vi "TTA_MATLAB_TxACPRTest.vi"(0 "Sub-Function Name":string, 1 "Instrument Cluster In":T3, 5 "Test Group":string, 11 "error in":errorcluster) -> (4 "SubTestSuccess":dbl[](array[numeric]), 12 "Instrument Cluster Out":T3, 15 "error out":errorcluster)   [LabVIEW 2016]
uses:
  TTA_Controls/TTA_Control_Complete_Settings_Cluster.ctl
  TTA_Controls/TTA_Control_Instrument_Cluster.ctl
  TTA_Globals/TTA_Global_Complete_Settings.vi
panel:
  out "Active ACPR Cluster":T1
  out "Channel":string
  out "Tx":string
  out "ACPR Results":T2(array[cluster])
  out "Test Status":string
  in  "Complete Settings Cluster":T4
  out "RFICs":i32[](array[numeric])
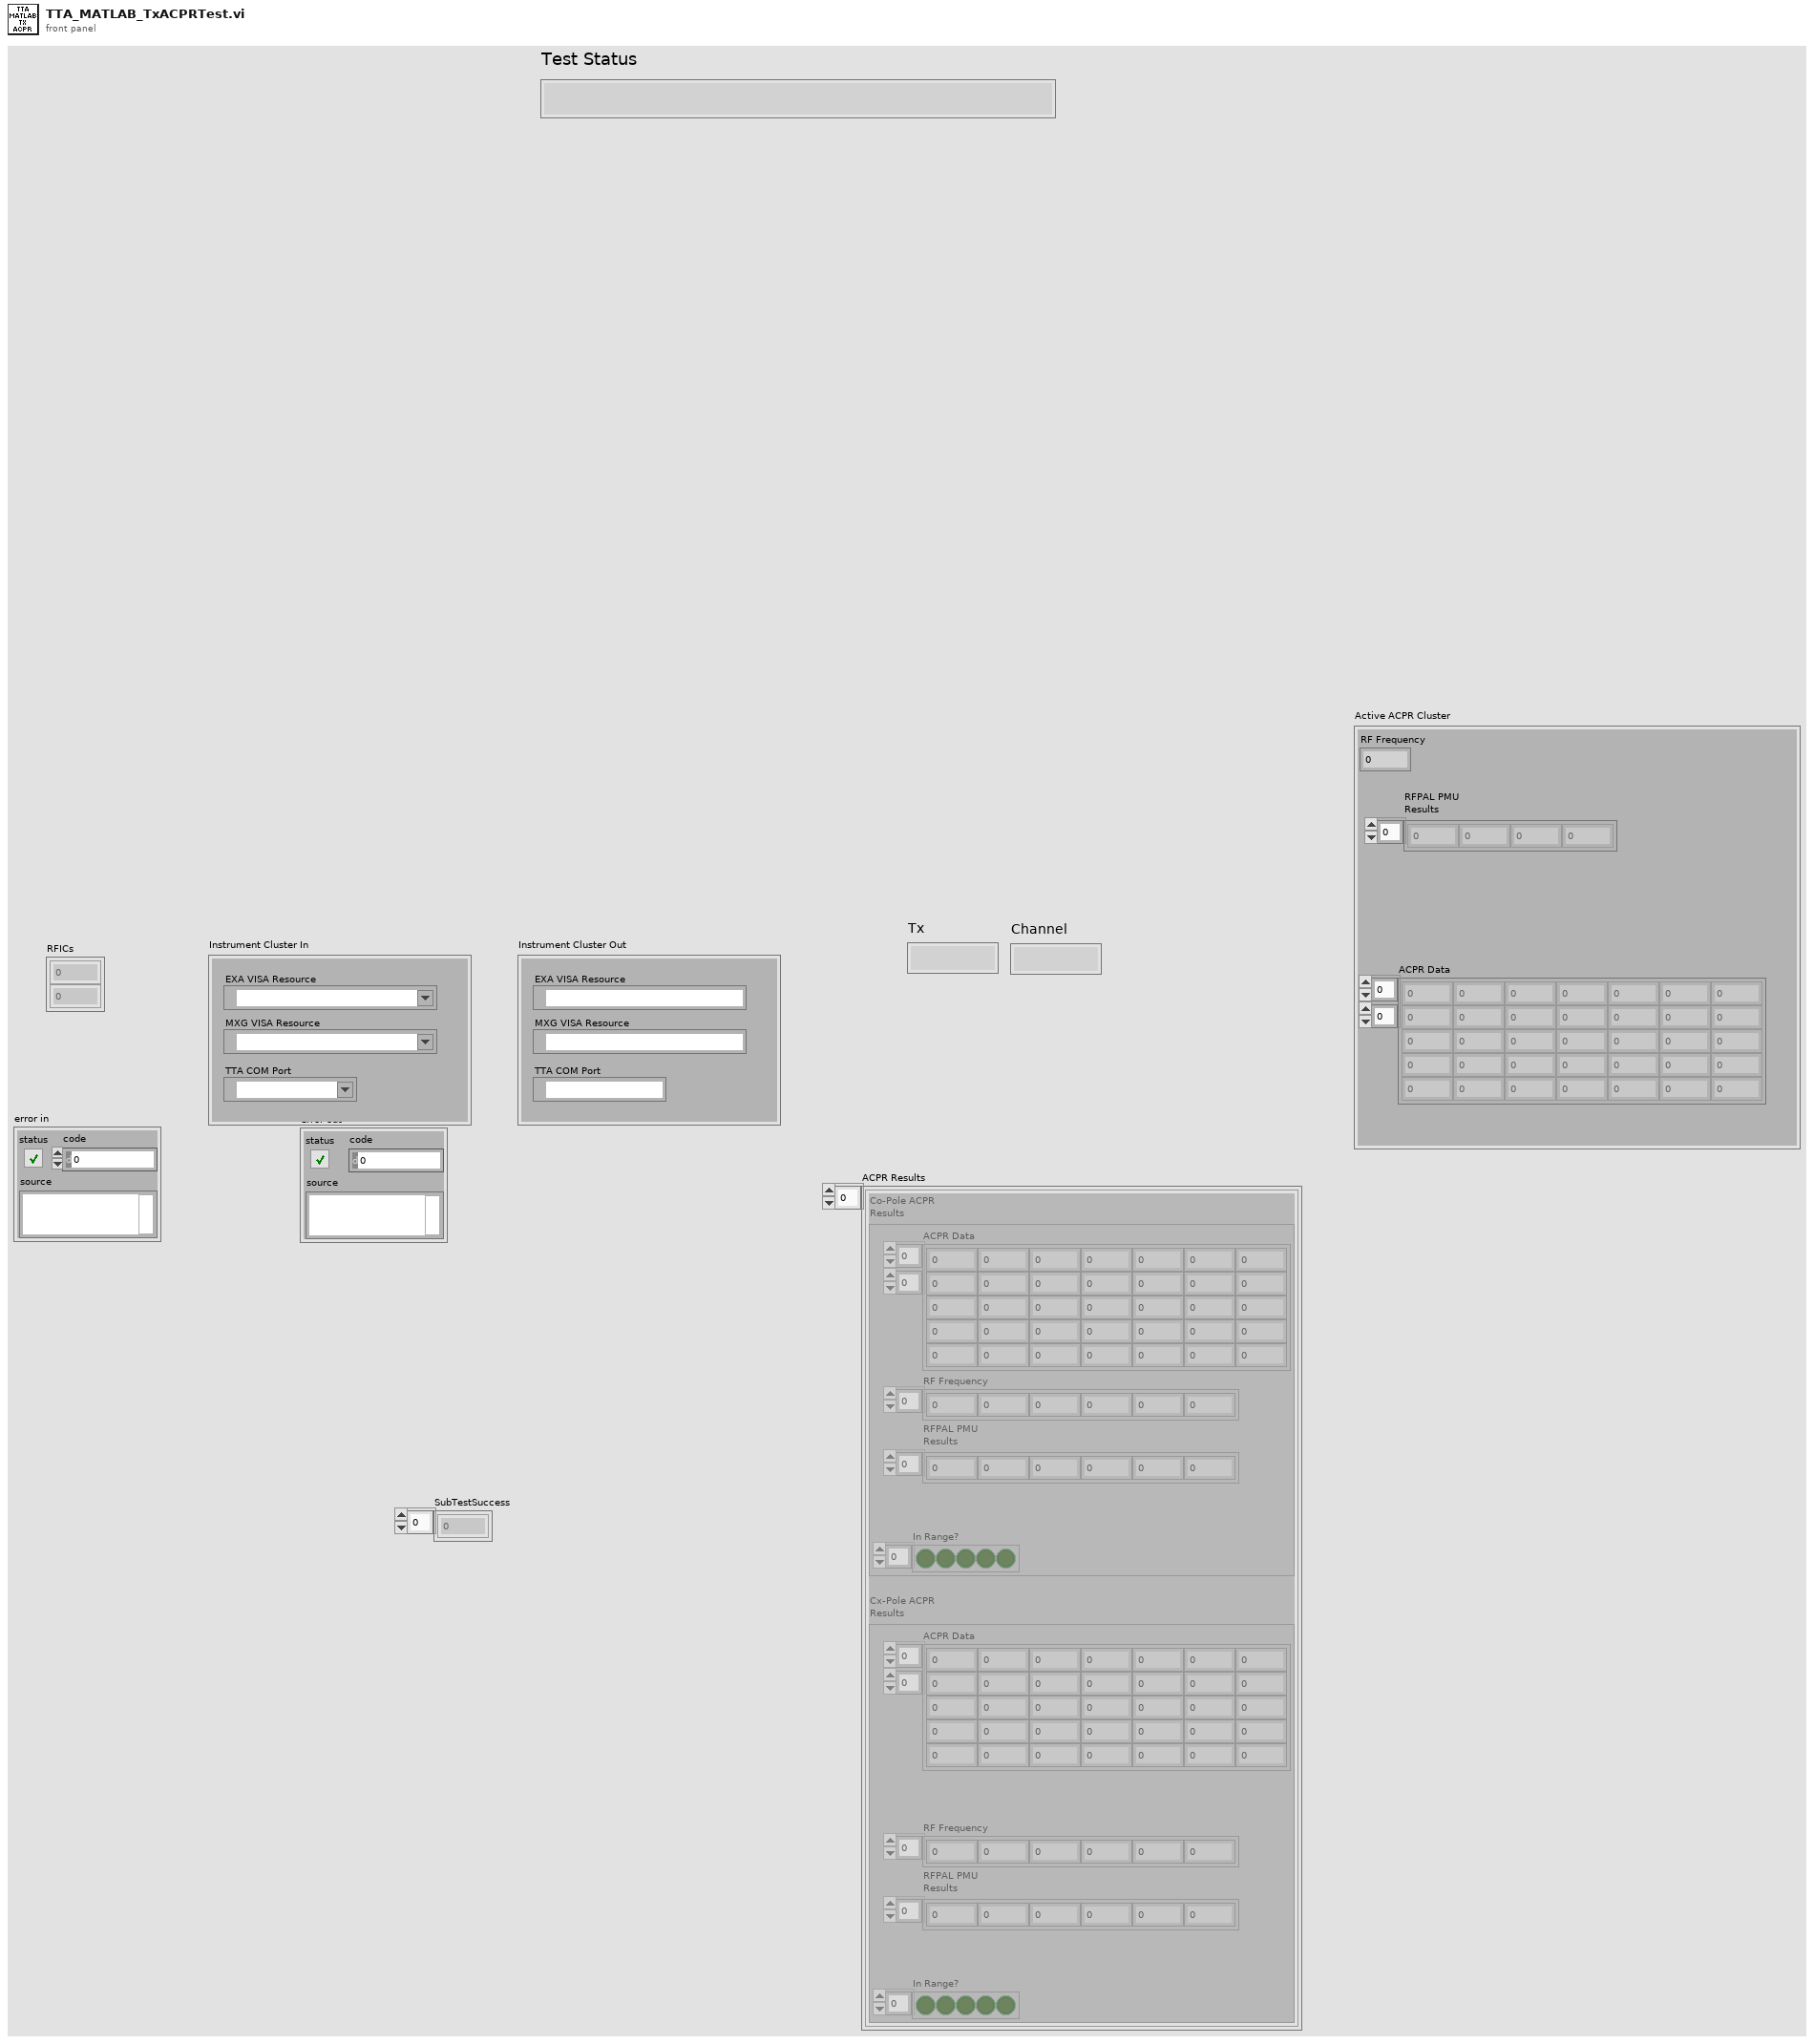
[diagram p1: front panel]
types:
  T1 = cluster{"RF Frequency":dbl, "RFPAL PMU\nResults":dbl[], "ACPR Data ":dbl[][]}
  T2 = cluster{"Co-Pole ACPR\nResults":cluster{"ACPR Data":dbl[][], "RF Frequency":dbl[], "RFPAL PMU\nResults":dbl[], "In Range?":bool[]}, "Cx-Pole ACPR\nResults":cluster{"ACPR Data":dbl[][], "RF Frequency":dbl[], "RFPAL PMU\nResults":dbl[], "In Range?":bool[]}}[]
  T3 = typedef "TTA_Control_Instrument_Cluster.ctl" = cluster{"EXA VISA Resource":refnum<visa-resource-name>, "MXG VISA Resource":refnum<visa-resource-name>, "TTA COM Port":refnum<visa-resource-name>}
  T4 = typedef "TTA_Control_Complete_Settings_Cluster.ctl" = cluster{"Brief Cluster":cluster{"STM Firmware File":string, "STM Firmware Address":string, "Required SW Version":string, "Template Used":string}, "Instrument Setting Cluster":cluster{"BDSFreq":dbl, "BDS Amp":dbl, "TxRFCal_Freq":dbl, "TxRFCal_Amp":dbl, "RxRFCal_Freq":dbl, "RxRFCal_Freq":dbl, "TxIF_Freq":dbl, "TxIF_Amp":dbl, "Tx_Output_Power_Signal_Freq":dbl, "Tx_ACPR_Signal_Freq":dbl, "Rx_RF_Freq":dbl, "Rx_RF_Amp":dbl, "Rx_Output_Power_Signal_Freq":dbl, "Rx_Output_Power_Sense_Freq":dbl}, "PAL Calibration\nInputs Cluster":cluster{"Amplitude Range\nMax(dBm)":dbl, "Amplitude Range\nMin(dBm)":dbl, "Amplitude Least\nCriteria (dBm)":dbl, "Frequency 1":dbl, "Frequency 2":dbl, "Frequency 3":dbl, "CAL Amplitude\nDecrement (dB)":dbl, "CAL Amplitude\nIncrement(dB)":dbl, "DownloadFile":string}, "TxOffset Cal Cluster":cluster{"Tx1 Offset (dB)":dbl, "Tx2 Offset (dB)":dbl, "Tx3 Offset (dB)":dbl, "Tx4 Offset (dB)":dbl, "Total RF Tx Loss (dB)":dbl}, "RxOffset Cal Cluster":cluster{"Rx1 Offset (dB)":dbl, "Rx2 Offset (dB)":dbl, "Rx3 Offset (dB)":dbl, "Rx4 Offset (dB)":dbl, "Total RF Rx Loss (dB)":dbl}, "TX Output Power Settings Cluster":cluster{"Frequency Sweep (MHz)":dbl[], "Sig Gen \nPower (dBm)":dbl, "Span (kHz)":dbl, "RBW (Hz)":dbl, "Ref Level (dBm)":dbl, "Low Power \nLimit":dbl, "High Power \nLimit":dbl, "DigAtt Max":dbl, "DigAtt Min":dbl}, "Tx ACPR Settings Cluster":cluster{"ACPR Filename":string, "Sampling Rate":dbl, "Power (dBm)":dbl, "IF Frequency Sweep (MHz)":dbl[], "State Name":string, "Mechanical\nAttenuation":dbl, "RefLevel Offset":dbl, "Amplitude Range\nMax (dBm)":dbl, "Amplitude Range\nMin (dBm)":dbl, "Cal Amp \nIncrement (dB)":dbl, "Cal Amp\nDecrement (dB)":dbl}, "Power Cal Cluster":cluster{"Power List (dBm)":dbl[], "Frequency (MHz)":dbl[], "Cal Decrement (dB)":dbl, "Cal Increment (dB)":dbl}, "Rx Received Power Settings Cluster":cluster{"Frequency Sweep (MHz)":dbl[], "Power (dBm)":dbl, "Span (kHz)":dbl, "RBW (Hz)":dbl, "Ref Level":dbl, "Low Power \nLimit (dBm)":dbl, "High Power\nLimit (dBm)":dbl}, "Tx Output Power Criteria Cluster":cluster{"CH1-TX1 \nMin":dbl, "CH1-TX1\nMax":dbl, "CH1-TXx3\nMin ":dbl, "CH1-TXx3\nMax":dbl, "CH2-TX1\nMin":dbl, "CH2-TX1\nMax":dbl, "CH2-TXx3\nMin":dbl, "CH2-TXx3\nMax":dbl}, "Tx ACPR Criteria Cluster":cluster{"Min Inband":dbl, "Max Close Outband":dbl, "Max Far Outband":dbl}, "Rx Output Power Criteria Cluster":cluster{"CH1-RX1 \nMin":dbl, "CH1-RX1 \nMax":dbl, "CH1-RXx3 \nMin":dbl, "CH1-RXx3\nMax":dbl, "CH2-RX1\nMin":dbl, "CH2-RX1\nMax":dbl, "CH2-RXx3\nMin":dbl, "CH2-RXx3\nMax":dbl}}
  T5 = cluster{"Amplitude Range\nMax(dBm)":dbl, "Amplitude Range\nMin(dBm)":dbl, "Amplitude Least\nCriteria (dBm)":dbl, "Frequency 1":dbl, "Frequency 2":dbl, "Frequency 3":dbl, "CAL Amplitude\nDecrement (dB)":dbl, "CAL Amplitude\nIncrement(dB)":dbl, "DownloadFile":string}
  T6 = cluster{"ACPR Filename":string, "Sampling Rate":dbl, "Power (dBm)":dbl, "IF Frequency Sweep (MHz)":dbl[], "State Name":string, "Mechanical\nAttenuation":dbl, "RefLevel Offset":dbl, "Amplitude Range\nMax (dBm)":dbl, "Amplitude Range\nMin (dBm)":dbl, "Cal Amp \nIncrement (dB)":dbl, "Cal Amp\nDecrement (dB)":dbl}
  T7 = cluster{"ACPR\nResults":cluster{"ACPR Data":dbl[][], "RF Frequency":dbl[], "RFPAL PMU\nResults":dbl[], "In Range?":bool[]}, "ACPR\nResults":cluster{"ACPR Data":dbl[][], "RF Frequency":dbl[], "RFPAL PMU\nResults":dbl[], "In Range?":bool[]}}[]
  T8 = cluster{"ACPR\nResults":cluster{"ACPR Data":dbl[][], "RF Frequency":dbl[], "RFPAL PMU\nResults":dbl[], "In Range?":bool[]}, "ACPR\nResults":cluster{"ACPR Data":dbl[][], "RF Frequency":dbl[], "RFPAL PMU\nResults":dbl[], "In Range?":bool[]}}
  T9 = cluster{"ACPR Data":dbl[][], "RF Frequency":dbl[], "RFPAL PMU\nResults":dbl[], "In Range?":bool[]}
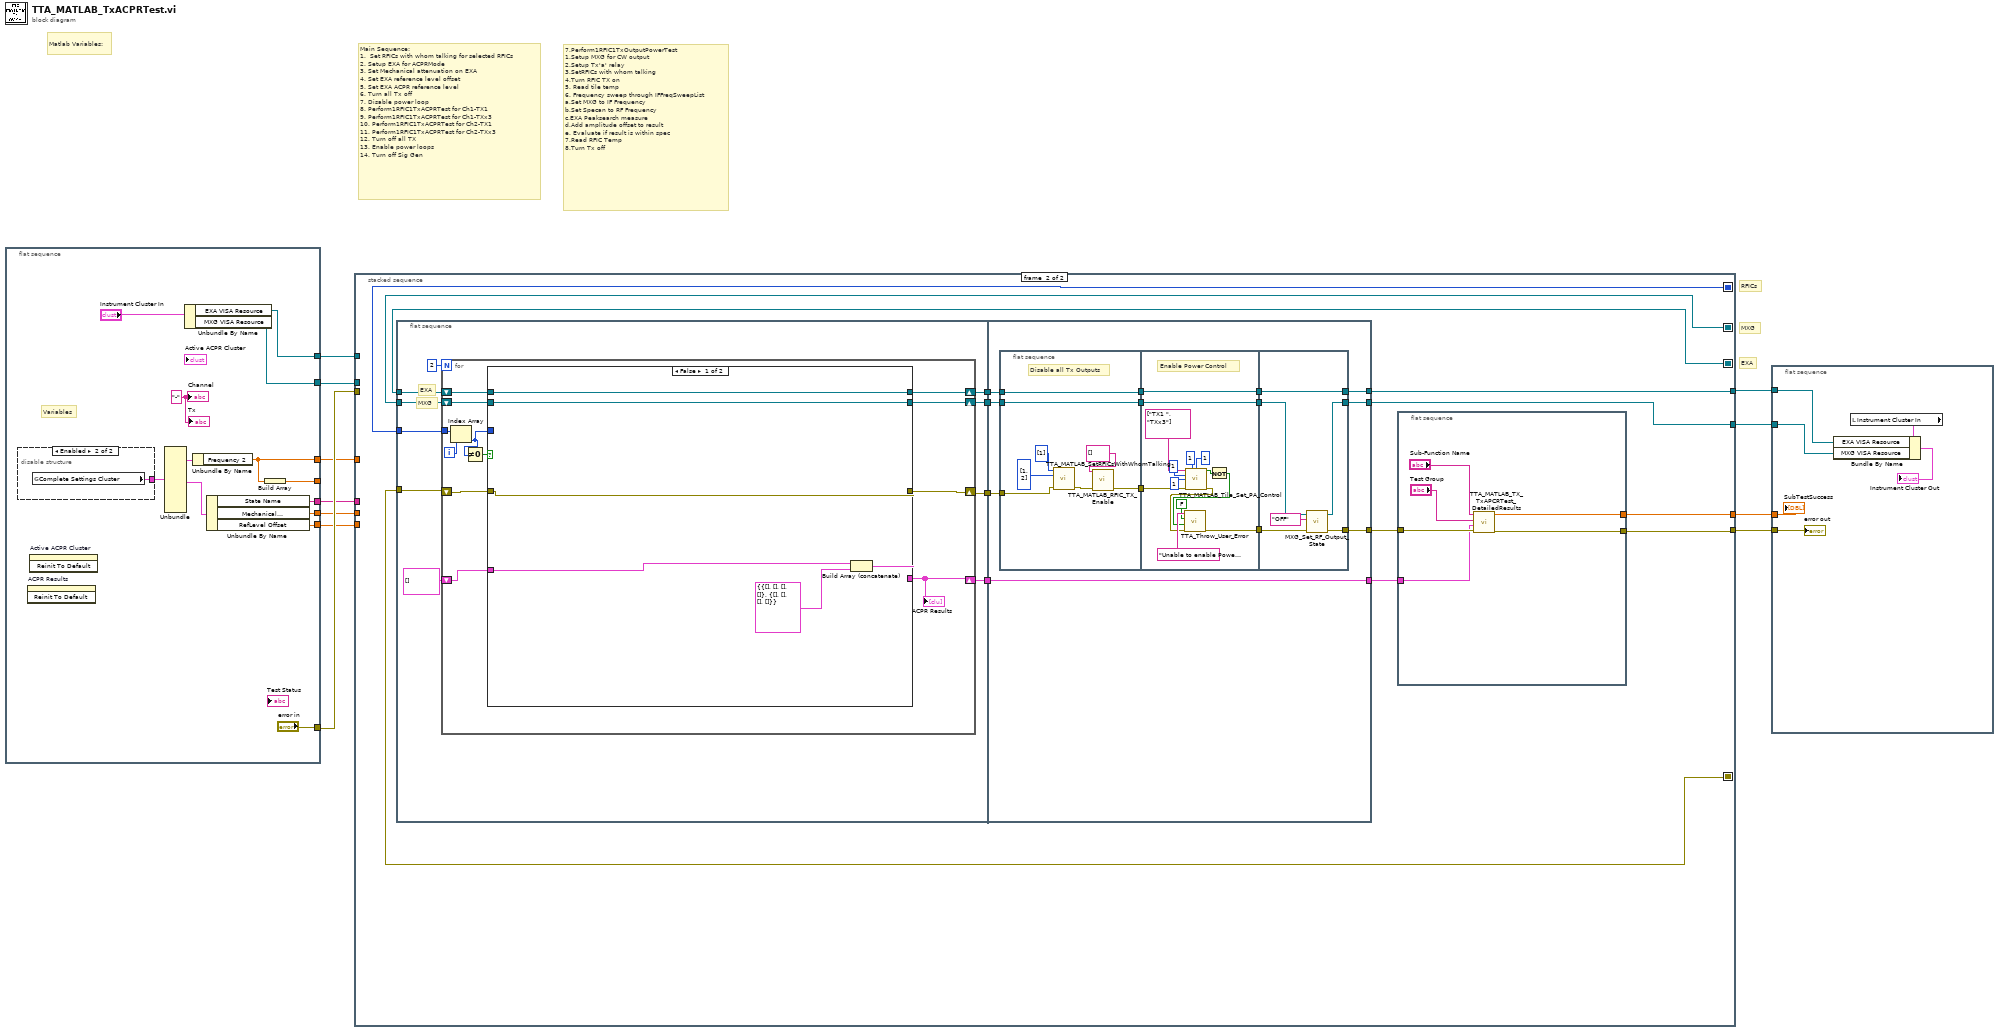
[diagram p0: block diagram]
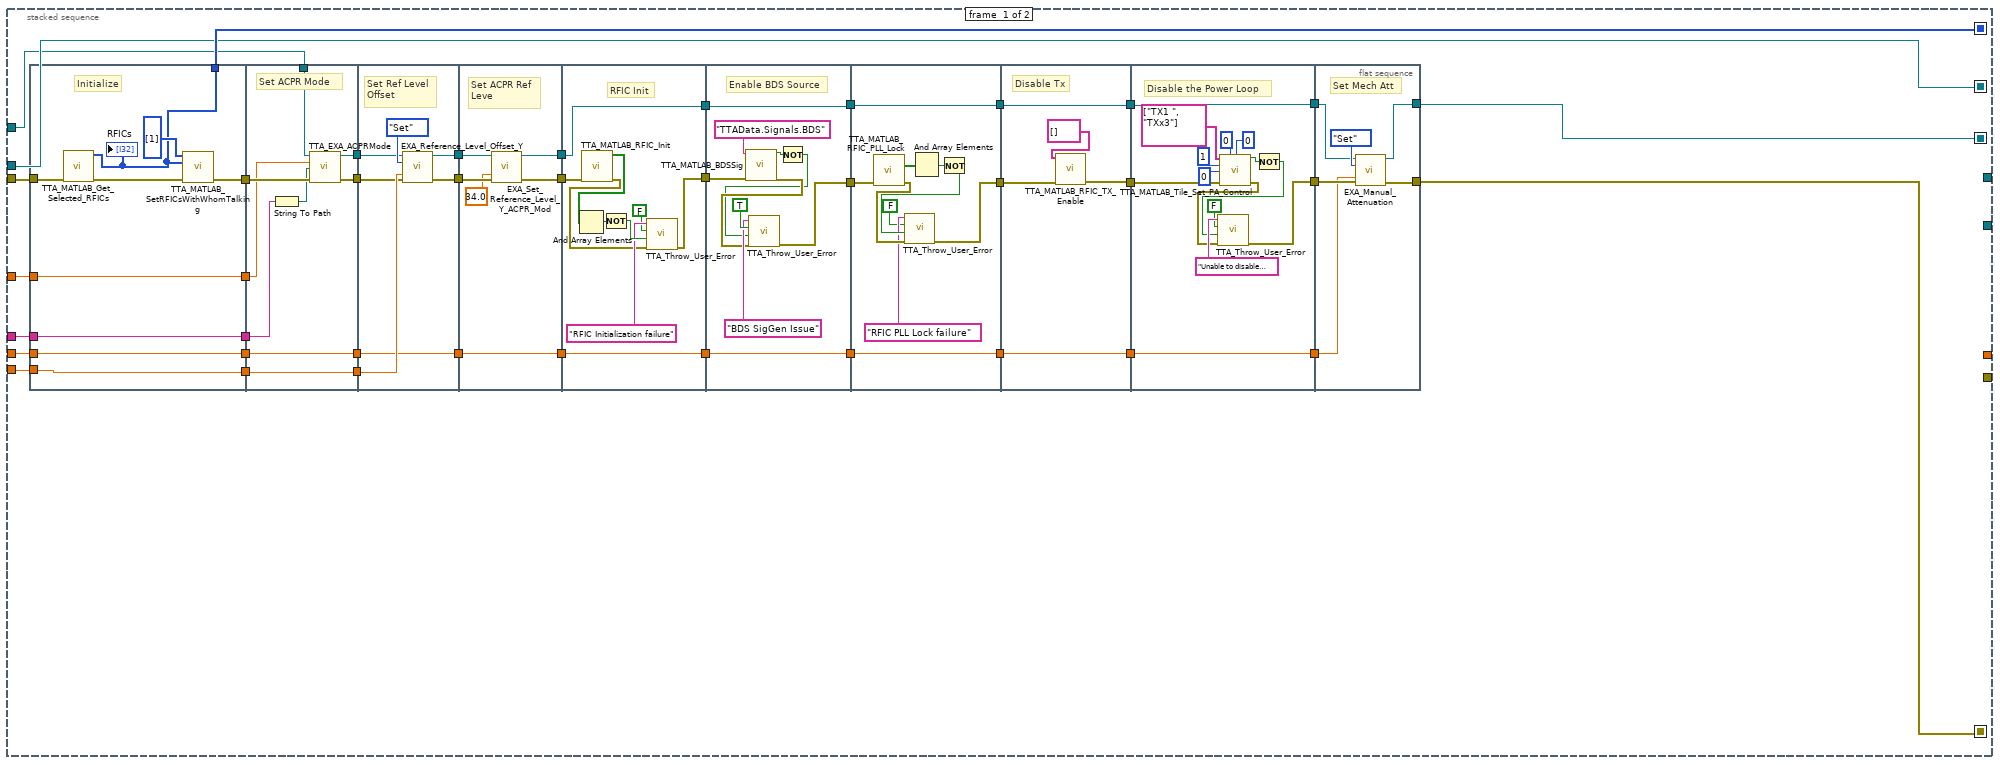
[diagram p2: hidden frame]
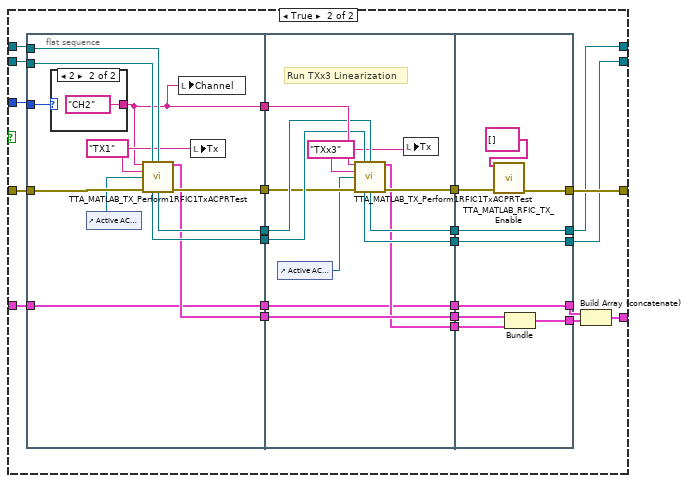
[diagram p3: hidden frame]
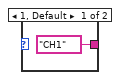
[diagram p4: hidden frame]
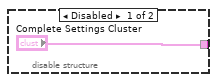
[diagram p5: hidden frame]
diagram:
  # "RFICs"
  # "EXA"
  # "MXG"
  # "Matlab Variables:"
  # "Main Sequence:\n1.  Set RFICs with whom talking for selected RFICs\n2. Setup EXA for ACPRMode\n3. Set Mechanical attenuation on EXA\n4. Set EXA reference level offset\n5. Set EXA ACPR reference level\n6. Turn all Tx off\n7. Disable power loop\n8. Perform1RFIC1TxACPRTest for Ch1-TX1\n9. Perform1RFIC1TxACPRTest for Ch1-TXx3\n10. Perform1RFIC1TxACPRTest for Ch2-TX1\n11. Perform1RFIC1TxACPRTest for Ch2-TXx3\n12. Turn off all TX\n13. Enable power loops\n14. Turn off Sig Gen"
  # "7.Perform1RFIC1TxOutputPowerTest\n1.Setup MXG for CW output\n2.Setup Tx'a' relay\n3.SetRFICs with whom talking\n4.Turn RFIC TX on\n5. Read tile temp\n6. Frequency sweep through IFFreqSweepList\na.Set MXG to IF Frequency\nb.Set Specan to RF Frequency\nc.EXA Peaksearch measure\nd.Add amplitude offset to result\ne. Evaluate if result is within spec\n7.Read RFIC Temp\n8.Turn Tx off"
  n1 = flat-sequence {
    tunnel: ["error in"] -> w11
    tunnel: [w19] -> w10
    tunnel: [w18] -> w9
    tunnel: [w22] -> _
    tunnel: [w17] -> w5
    tunnel: [w15] -> w4
    tunnel: [w14] -> w3
    tunnel: [w13] -> w2
    frame #0 {
      w12 = "-" ("Channel")
      # "Variables"
      n2 = disable-structure shown="Enabled" {
        disable-tunnel: ["Complete Settings Cluster" w26] -> w24
        frame Disabled {
        }
        frame Enabled {
          n3 = global read "TTA_Global_Complete_Settings.vi" "Complete Settings Cluster"() -> (w26:T4)
        }
      }
      n4 = invoke on="ACPR Results" class="Arr (strict)" method="Reinit To Default"() -> ()  [unwired: 3 in, 3 out]
      n5 = invoke on="Active ACPR Cluster" class="Clust (strict)" method="Reinit To Default"() -> ()  [unwired: 3 in, 3 out]
      n6 = Unbundle(w24) -> ("PAL Calibration\nInputs Cluster"=w21:T5, "Tx ACPR Settings Cluster"=w16:T6)  [unwired: 10 out]
      n7 = Unbundle By Name("Instrument Cluster In") -> ("EXA VISA Resource"=w19:refnum<visa-resource-name>, "MXG VISA Resource"=w18:refnum<visa-resource-name>)
      n8 = Unbundle By Name(w21) -> ("Frequency 2"=w17:dbl)
      n9 = Unbundle By Name(w16) -> ("State Name"=w15:string, "Mechanical\nAttenuation"=w14:dbl, "RefLevel Offset"=w13:dbl)
      n10 = Build Array(w17) -> (w22:dbl[])
      "Channel" <- w12
      "Tx" <- w12
    }
  }
  n11 = stacked-sequence {
    seq-local: [w65 _] -> [_ w166]
    seq-local: [w44 _] -> [_ w164]
    seq-local: [w57 _] -> [_ w165]
    seq-local: [w62 _] -> [_ w163]
    tunnel: w11 -> [w66 _]
    tunnel: w10 -> [w59 _]
    tunnel: w9 -> [w62 _]
    tunnel: [_ w154] -> w8
    tunnel: [_ w160] -> w7
    tunnel: [_ w159] -> w6
    tunnel: w5 -> [w61 _]
    tunnel: w4 -> [w56 _]
    tunnel: w3 -> [w54 _]
    tunnel: w2 -> [w52 _]
    tunnel: [_ w153] -> w1
    frame #0 {
      n12 = flat-sequence {
        tunnel: w66 -> [w73]
        tunnel: [w72] -> w65
        tunnel: [w71] -> w64
        tunnel: w61 -> [w70]
        tunnel: [w70] -> w60
        tunnel: w56 -> [w69]
        tunnel: [w69] -> w55
        tunnel: w54 -> [w68]
        tunnel: [w68] -> w53
        tunnel: w52 -> [w67]
        tunnel: [w67] -> w51
        tunnel: w64 -> [w84]
        tunnel: w60 -> [w82]
        tunnel: w59 -> [w83]
        tunnel: w55 -> [w81]
        tunnel: w53 -> [w76]
        tunnel: [w79] -> w30
        tunnel: w51 -> [w79]
        tunnel: [w78] -> w29
        tunnel: [w77] -> w28
        tunnel: [w76] -> w27
        tunnel: [w88] -> w50
        tunnel: [w89] -> w48
        tunnel: w30 -> [w91]
        tunnel: [w85] -> w31
        tunnel: w29 -> [w87]
        tunnel: w28 -> [w86]
        tunnel: w27 -> [w85]
        tunnel: w50 -> [w97]
        tunnel: [w94] -> w49
        tunnel: w48 -> [w96]
        tunnel: [w95] -> w47
        tunnel: [w92] -> w32
        tunnel: w31 -> [w92]
        tunnel: w49 -> [w102]
        tunnel: [w100] -> w63
        tunnel: w47 -> [w99]
        tunnel: [w99] -> w58
        tunnel: [w98] -> w33
        tunnel: w32 -> [w98]
        tunnel: w63 -> [w113]
        tunnel: w58 -> [w110]
        tunnel: [w110] -> w43
        tunnel: [w109] -> w41
        tunnel: [w108] -> w34
        tunnel: w33 -> [w108]
        tunnel: w43 -> [w127]
        tunnel: [w127] -> w42
        tunnel: w41 -> [w120]
        tunnel: [w119] -> w40
        tunnel: [w118] -> w35
        tunnel: w34 -> [w118]
        tunnel: w42 -> [w132]
        tunnel: [w132] -> w46
        tunnel: [w129] -> w45
        tunnel: w40 -> [w130]
        tunnel: [w128] -> w36
        tunnel: w35 -> [w128]
        tunnel: w46 -> [w137]
        tunnel: w45 -> [w136]
        tunnel: [w137] -> w39
        tunnel: [w134] -> w38
        tunnel: [w133] -> w37
        tunnel: w36 -> [w133]
        tunnel: [w151] -> w44
        tunnel: [w148] -> w57
        tunnel: w39 -> [w149]
        tunnel: w38 -> [w152]
        tunnel: w37 -> [w147]
        frame #0 {
          # "Initialize"
          n13 = call "TTA_MATLAB_Get_Selected_RFICs.vi"("error in"=w73) -> ("RFICs"=w72:i32[], "error out"=w74:errorcluster)  [unwired: 13 in]
          "RFICs" <- w72
          n14 = call "TTA_MATLAB_SetRFICsWithWhomTalking.vi"("Panel Array"=i32[] [1], "RFIC Array"=w72, "error in"=w74) -> ("error out"=w71:errorcluster)  [unwired: 12 in]
        }
        frame #1 {
          # "Set ACPR Mode"
          n15 = String To Path(string=w81) -> (path=w80:path)
          n16 = call "TTA_EXA_ACPRMode.vi"("VISA resource In"=w83, "Frequency (MHz)"=w82, "State File"=w80, "error in"=w84) -> ("VISA resource Out"=w77:refnum<visa-resource-name>, "error out"=w78:errorcluster)  [unwired: 10 in]
        }
        frame #2 {
          # "Set Ref Level \nOffset"
          n17 = call "EXA_Reference_Level_Offset_Y.vi"("VISA resource name"=w86, "Mode"=enum16{"Set", "Get"}."Set", "Reference Level \nOffset (dBm)"=w91, "error in"=w87) -> ("VISA resource name"=w89:refnum<visa-resource-name>, "error out"=w88:errorcluster)  [unwired: 9 in, 1 out]
        }
        frame #3 {
          # "Set ACPR Ref\nLeve"
          n18 = call "EXA_Set_Reference_Level_Y_ACPR_Mod.vi"("VISA resource name"=w96, "Reference Level \nOffset (dBm)"=34.0 ("Reference Level \nOffset (dBm)"), "error in"=w97) -> ("VISA resource name"=w95:refnum<visa-resource-name>, "error out"=w94:errorcluster)  [unwired: 11 in]
        }
        frame #4 {
          # "RFIC Init"
          n19 = call "TTA_MATLAB_RFIC_Init.vi"("error in"=w102) -> ("SuccessComm"=w107:bool[], "error out"=w101:errorcluster)  [unwired: 13 in]
          n20 = And Array Elements(Boolean array=w107) -> (logical AND=w106:bool)
          n21 = Not(x=w106) -> (.not. x?=w105:bool)
          n22 = call "TTA_Throw_User_Error.vi"("error in"=w101, "Error?"=w105, "Stop Execution on Fail"=FALSE, "Error Message"="RFIC Initialization failure") -> ("error out"=w100:errorcluster)  [unwired: 7 in]
        }
        frame #5 {
          # "Enable BDS Source"
          n23 = call "TTA_MATLAB_BDSSig.vi"("Signal Settings"="TTAData.Signals.BDS", "error in"=w113) -> ("Success"=w114:bool, "error out"=w112:errorcluster)  [unwired: 12 in]
          n24 = Not(x=w114) -> (.not. x?=w111:bool)
          n25 = call "TTA_Throw_User_Error.vi"("error in"=w112, "Error?"=w111, "Stop Execution on Fail"=TRUE, "Error Message"="BDS SigGen Issue") -> ("error out"=w109:errorcluster)  [unwired: 7 in]
        }
        frame #6 {
          n26 = call "TTA_MATLAB_RFIC_PLL_Lock.vi"("error in"=w120) -> ("SuccessComm"=w121:bool[], "error out"=w126:errorcluster)  [unwired: 11 in, 2 out]
          n27 = And Array Elements(Boolean array=w121) -> (logical AND=w124:bool)
          n28 = Not(x=w124) -> (.not. x?=w125:bool)
          n29 = call "TTA_Throw_User_Error.vi"("error in"=w126, "Error?"=w125, "Stop Execution on Fail"=FALSE, "Error Message"="RFIC PLL Lock failure") -> ("error out"=w119:errorcluster)  [unwired: 7 in]
        }
        frame #7 {
          # "Disable Tx"
          n30 = call "TTA_MATLAB_RFIC_TX_Enable.vi"("Channels"=string[] [], "error in"=w130) -> ("error out"=w129:errorcluster)  [unwired: 12 in, 1 out]
        }
        frame #8 {
          # "Disable the Power Loop"
          n31 = call "TTA_MATLAB_Tile_Set_PA_Control.vi"("Channels"=string[] ["TX1 ", "TXx3"], "OutPower"=0, "InPower"=0, "Temp"=1, "Current"=0, "error in"=w136) -> ("Success"=w140:bool, "error out"=w138:errorcluster)  [unwired: 6 in, 2 out]
          n32 = Not(x=w140) -> (.not. x?=w139:bool)
          n33 = call "TTA_Throw_User_Error.vi"("error in"=w138, "Error?"=w139, "Stop Execution on Fail"=FALSE, "Error Message"="Unable to disable Power Loop") -> ("error out"=w134:errorcluster)  [unwired: 7 in]
        }
        frame #9 {
          # "Set Mech Att"
          n34 = call "EXA_Manual_Attenuation.vi"("VISA resource name"=w149, "Mode"=enum16{"Set", "Get"}."Set", "Attenuation (dB)"=w147, "error in"=w152) -> ("VISA resource name"=w148:refnum<visa-resource-name>, "error out"=w151:errorcluster)  [unwired: 9 in, 1 out]
        }
      }
    }
    frame #1 {
      n35 = flat-sequence {
        tunnel: w166 -> [w180]
        tunnel: w165 -> [w182]
        tunnel: w163 -> [w181]
        tunnel: w164 -> [w179]
        tunnel: [w177] -> w162
        tunnel: [w176] -> w161
        tunnel: [w178] -> w158
        tunnel: [w173] -> w156
        tunnel: w162 -> [w270]
        tunnel: w161 -> [w269]
        tunnel: [w262] -> w157
        tunnel: [w261] -> w160
        tunnel: [w260] -> w159
        tunnel: w158 -> [w271]
        tunnel: w156 -> [w259]
        tunnel: [w259] -> w155
        frame #0 {
          # "EXA"
          # "MXG"
          n36 = for {
            N: 2 -> [_]
            tunnel: w180 -> [w186]
            shift-right: [w191] -> w178
            shift-left: w179 -> [w192]
            shift-right: [w190] -> w177
            shift-left: w182 -> [w194]
            shift-right: [w189] -> w176
            shift-left: w181 -> [w193]
            shift-right: [w187] -> w173
            shift-left: T7 [] -> [w188]
            i -> [w185]
            n37 = Index Array(array=w186, index=w185) -> (element=w183:i32)
            n38 = Not Equal To 0?(x=w183) -> (x != 0?=w184:bool)
            n39 = case shown="False" w184 {
              tunnel: w194 -> [w200 w211]
              tunnel: w193 -> [w199 w210]
              tunnel: w183 -> [_ w209]
              tunnel: w192 -> [w198 w208]
              tunnel: [w198 w207] -> w191
              tunnel: [w200 w206] -> w190
              tunnel: [w199 w205] -> w189
              tunnel: w188 -> [w197 w203]
              tunnel: [w196 w201] -> w187
              frame False {
                n40 = Build Array (concatenate)(w197, T8 {"ACPR\nResults"={"ACPR Data"=[], "RF Frequency"=[], "RFPAL PMU\nResults"=[], "In Range?"=[]}, "ACPR\nResults"={"ACPR Data"=[], "RF Frequency"=[], "RFPAL PMU\nResults"=[], "In Range?"=[]}} ("output cluster")) -> (w196:T7)
              }
              frame True {
                n41 = flat-sequence {
                  tunnel: w209 -> [w235]
                  tunnel: w211 -> [w234]
                  tunnel: w210 -> [w233]
                  tunnel: w208 -> [w232]
                  tunnel: [w226] -> w223
                  tunnel: [w231] -> w222
                  tunnel: [w230] -> w221
                  tunnel: [w229] -> w220
                  tunnel: [w228] -> w219
                  tunnel: w203 -> [w225]
                  tunnel: [w225] -> w218
                  tunnel: w223 -> [w249]
                  tunnel: w222 -> [w247]
                  tunnel: w221 -> [w246]
                  tunnel: [w248] -> w217
                  tunnel: [w245] -> w216
                  tunnel: [w244] -> w215
                  tunnel: w220 -> [w243]
                  tunnel: [w242] -> w214
                  tunnel: w219 -> [w242]
                  tunnel: [w241] -> w213
                  tunnel: w218 -> [w239]
                  tunnel: [w239] -> w212
                  tunnel: [w257] -> w206
                  tunnel: [w258] -> w205
                  tunnel: w217 -> [w255]
                  tunnel: w216 -> [w258]
                  tunnel: w215 -> [w257]
                  tunnel: [w254] -> w207
                  tunnel: w214 -> [w253]
                  tunnel: w213 -> [w252]
                  tunnel: [w251] -> w204
                  tunnel: w212 -> [w250]
                  tunnel: [w250] -> w202
                  frame #0 {
                    w227 = "TX1" ("Tx")
                    n42 = case shown="2" w235 {
                      tunnel: ["CH1" ("Channel") "CH2" ("Channel")] -> w226
                      frame 1, Default {
                      }
                      frame 2 {
                      }
                    }
                    n43 = control-ref of="Active ACPR Cluster"() -> (w224:refnum<vi>)
                    n44 = call "TTA_MATLAB_TX_Perform1RFIC1TxACPRTest.vi"("Channel"=w226, "MXG VISA Resource In"=w233, "EXA VISA Resource"=w234, "Tx"=w227, "Active ACPR Refnum"=w224, "error in"=w232) -> ("ACPR\nResults"=w228:T9, "MXG VISA Resource Out"=w231:refnum<visa-resource-name>, "EXA VISA Resource Out"=w230:refnum<visa-resource-name>, "error out"=w229:errorcluster)  [unwired: 6 in]
                    n45 = local write "Channel"(w226) -> ()
                    n46 = local write "Tx"(w227) -> ()
                  }
                  frame #1 {
                    w240 = "TXx3" ("Tx")
                    # "Run TXx3 Linearization"
                    n47 = control-ref of="Active ACPR Cluster"() -> (w238:refnum<vi>)
                    n48 = call "TTA_MATLAB_TX_Perform1RFIC1TxACPRTest.vi"("Channel"=w249, "MXG VISA Resource In"=w247, "EXA VISA Resource"=w246, "Tx"=w240, "Active ACPR Refnum"=w238, "error in"=w243) -> ("ACPR\nResults"=w241:T9, "MXG VISA Resource Out"=w245:refnum<visa-resource-name>, "EXA VISA Resource Out"=w244:refnum<visa-resource-name>, "error out"=w248:errorcluster)  [unwired: 6 in]
                    n49 = local write "Tx"(w240) -> ()
                  }
                  frame #2 {
                    n50 = call "TTA_MATLAB_RFIC_TX_Enable.vi"("Channels"=string[] [], "error in"=w255) -> ("error out"=w254:errorcluster)  [unwired: 12 in, 1 out]
                    n51 = Bundle("ACPR\nResults"=w253, "ACPR\nResults"=w252) -> (w251:T8)  [unwired: 1 in]
                  }
                }
                n52 = Build Array (concatenate)(w202, w204) -> (w201:T7)
              }
            }
            "ACPR Results" <- w187
          }
        }
        frame #1 {
          n53 = flat-sequence {
            tunnel: w271 -> [w277]
            tunnel: w270 -> [w273]
            tunnel: w269 -> [w272]
            tunnel: [w274] -> w268
            tunnel: [w273] -> w267
            tunnel: [w272] -> w266
            tunnel: w268 -> [w282]
            tunnel: w267 -> [w293]
            tunnel: w266 -> [w292]
            tunnel: [w293] -> w265
            tunnel: [w292] -> w264
            tunnel: [w280] -> w263
            tunnel: [w296] -> w261
            tunnel: [w299] -> w260
            tunnel: w265 -> [w299]
            tunnel: w264 -> [w297]
            tunnel: w263 -> [w298]
            tunnel: [w294] -> w262
            frame #0 {
              # "Disable all Tx Outputs"
              n54 = call "TTA_MATLAB_SetRFICsWithWhomTalking.vi"("Panel Array"=i32[] [1], "RFIC Array"=i32[] [1, 2], "error in"=w277) -> ("error out"=w275:errorcluster)  [unwired: 12 in]
              n55 = call "TTA_MATLAB_RFIC_TX_Enable.vi"("Channels"=string[] [], "error in"=w275) -> ("error out"=w274:errorcluster)  [unwired: 12 in, 1 out]
            }
            frame #1 {
              # "Enable Power Control"
              n56 = call "TTA_MATLAB_Tile_Set_PA_Control.vi"("Channels"=string[] ["TX1 ", "TXx3"], "OutPower"=1, "InPower"=1, "Temp"=1, "Current"=1, "error in"=w282) -> ("Success"=w285:bool, "error out"=w283:errorcluster)  [unwired: 6 in, 2 out]
              n57 = Not(x=w285) -> (.not. x?=w284:bool)
              n58 = call "TTA_Throw_User_Error.vi"("error in"=w283, "Error?"=w284, "Stop Execution on Fail"=FALSE, "Error Message"="Unable to enable Power Loop") -> ("error out"=w280:errorcluster)  [unwired: 7 in]
            }
            frame #2 {
              n59 = call "MXG_Set_RF_Output_State.vi"("error in"=w298, "RF Output State"="OFF", "VISA resource name"=w297) -> ("error out"=w294:errorcluster, "VISA resource name"=w296:refnum<visa-resource-name>)  [unwired: 7 in]
            }
          }
        }
      }
      n60 = flat-sequence {
        tunnel: w157 -> [w172]
        tunnel: w155 -> [w171]
        tunnel: [w168] -> w154
        tunnel: [w167] -> w153
        frame #0 {
          n61 = call "TTA_MATLAB_TX_TxAPCRTest_DetailedResults.vi"("error in"=w172, "ACPR Results"=w171, "TestGroup"="Test Group", "SubTest"="Sub-Function Name") -> ("error out"=w168:errorcluster, "SubTestSuccess"=w167:dbl[])  [unwired: 6 in]
        }
      }
    }
  }
  n62 = flat-sequence {
    tunnel: w8 -> [w305]
    tunnel: w7 -> [w302]
    tunnel: w6 -> [w303]
    tunnel: w1 -> [w300]
    frame #0 {
      n63 = local read "Instrument Cluster In"() -> (w301:T3)
      n64 = Bundle By Name(cluster=w301, "EXA VISA Resource"=w303, "MXG VISA Resource"=w302) -> (→"Instrument Cluster Out":T3)
      "error out" <- w305
      "SubTestSuccess" <- w300
    }
  }
